vi "1. CoffeeMaker Front Panel.vi"() -> ()   [LabVIEW 2018]
doc: "Coffee Machine Version 1.0: only front panel"
panel:
  in  "Power Switch":bool
  in  "Simulation":cluster{"Water":dbl, "Coffee":dbl, "Milk":dbl} {"Milk" scale=0.0..100.0; "Water" scale=0.0..100.0; "Coffee" scale=0.0..100.0}
  out "Display":T1 {"Coffee" scale=0.0..80.0; "Brewing Chamber" scale=0.0..80.0}
  in  "Control Elements":T2 {"Type" min=0 max=2 scale=0.0..2.0}
  # "Coffee Selection"
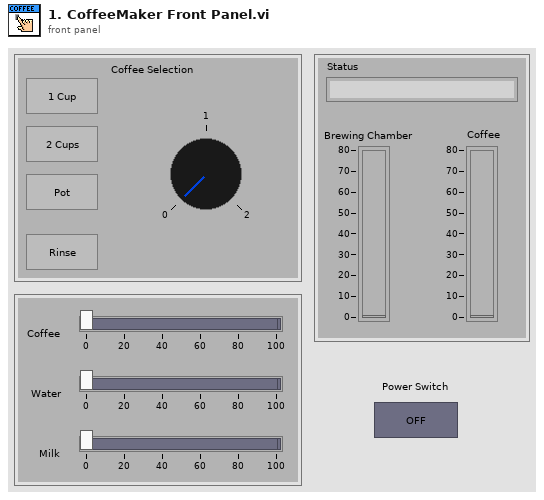
[diagram p1: front panel]
types:
  T1 = cluster{"Brewing Chamber":dbl, "Coffee":dbl, "Status":string}
  T2 = cluster{"1 Cup":bool, "2 Cups":bool, "Pot":bool, "Rinse":bool, "Type":i8}
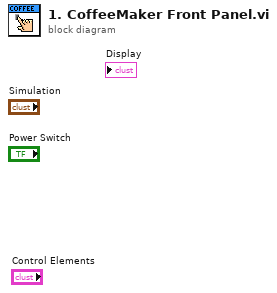
[diagram p0: block diagram]
diagram:
